vi "Vision Research Phantom Series Default Instrument Setup.vi"(11 "Error In (no error)":errorcluster) -> (15 "Error Out":errorcluster)   [LabVIEW 2013, in "VRI.lvlib"]
doc: "This Utility VI is part of the standard National Instruments driver requirements and would send a default command string to the instrument whenever a new VISA session is opened if the command were supported. This VI is intended to be used as a subVI for the Vision Research Phantom Series Initialize and Vision Research Phantom Series Reset VI's. Altering this VI could cause these two VI's to operate incorrectly. If a default command is to be implemented, show the true case on the diagram, right click on the case structure and select remove case structure, and enter the command string.\n\nWritten by:\nBLOOMY CONTROLS, INC\nWINDSOR, CT 06095, USA\n860-298-9925\nwww.bloomy.com\nV1.0.0\nMay, 2004"
uses:
  VRI.lvlib
panel:
  in  "Case Constant\n(See Context Help)":bool
  # "For instructions on the use of this VI, press Ctrl+H to display the help window and move the mouse over the icon, controls, and indicators"
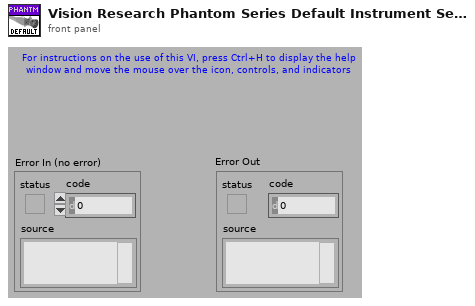
[diagram p1: front panel]
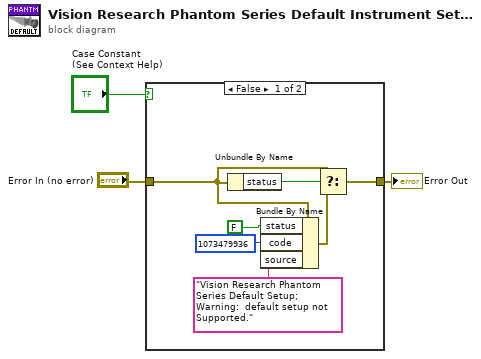
[diagram p0: block diagram]
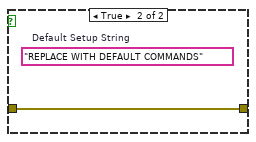
[diagram p2: hidden frame]
diagram:
  n1 = case shown="False" "Case Constant\n(See Context Help)" {
    tunnel: "Error In (no error)" -> [w5 w11]
    tunnel: [w4 w11] -> w2
    frame False {
      n2 = Unbundle By Name(w5) -> ("status"=w7:bool)
      n3 = Bundle By Name(cluster=w5, "status"=FALSE, "code"=1073479936, "source"="Vision Research Phantom Series Default Setup; Warning:  default setup not Supported.") -> (w6:errorcluster)
      n4 = Select(t=w5, s=w7, f=w6) -> (s? t:f=w4:errorcluster)
    }
    frame True {
      (unwired) "REPLACE WITH DEFAULT COMMANDS"  # Default Setup String
    }
  }
  "Error Out" <- w2
